vi "Bool to Boolean String.vi"(1 "bool":bool) -> (0 "boolean string":string)   [LabVIEW 2017]
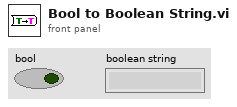
[diagram p1: front panel]
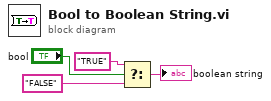
[diagram p0: block diagram]
diagram:
  n1 = Select(t="TRUE", s="bool", f="FALSE") -> (s? t:f=→"boolean string":string)
